vi "Insight Float Package.vi"(1 "Decimal Places":i32=2, 2 "Footer":string, 3 "Float":dbl format="%#_2f", 4 "Header":string) -> (0 "resulting string":string)   [LabVIEW 2013]
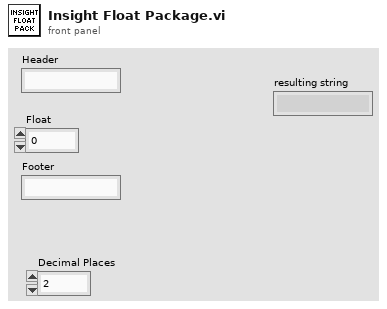
[diagram p1: front panel]
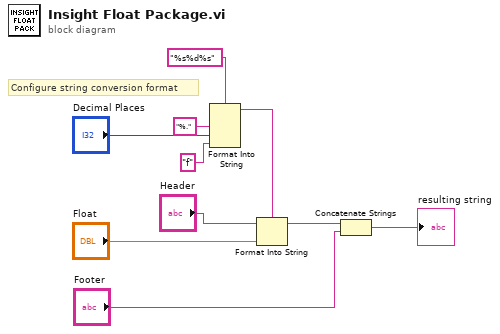
[diagram p0: block diagram]
diagram:
  # "Configure string conversion format"
  n1 = Format Into String(format string="%s%d%s", "%." ("string"), "Decimal Places", "f" ("string")) -> (resulting string=w8:string)  [unwired: 2 in, 1 out]
  n2 = Format Into String(format string=w8, initial string="Header", "Float") -> (resulting string=w3:string)  [unwired: 1 in, 1 out]
  n3 = Concatenate Strings(w3, "Footer") -> (→"resulting string":string)
